vi "Record.vi"(7 "Station":string, 8 "InputResult":string, 9 "NGCode":string, 10 "PN":string, 11 "SN":string) -> (3 "Result":string)   [LabVIEW 2020]
uses:
  <vilib>/Utility/config.llb/Read Key (String).vi
  <vilib>/Utility/config.llb/Read Key (I32).vi
  <vilib>/Utility/config.llb/Write Key (String).vi
  <vilib>/Utility/config.llb/Write Key (I32).vi
  <vilib>/Utility/config.llb/NI_LVConfig.lvlib
panel:
  out "appended path":path
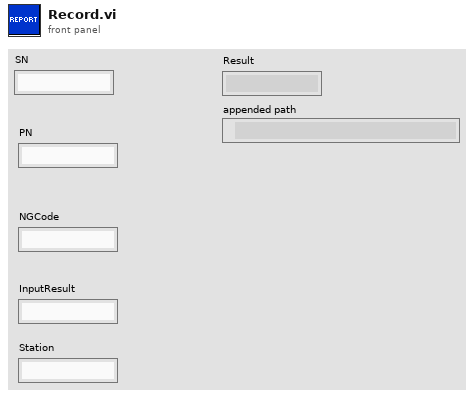
[diagram p1: front panel]
types:
  T1 = typedef "NI_LVConfig.lvlib/Config Data RefNum.ctl" = refnum<k1>
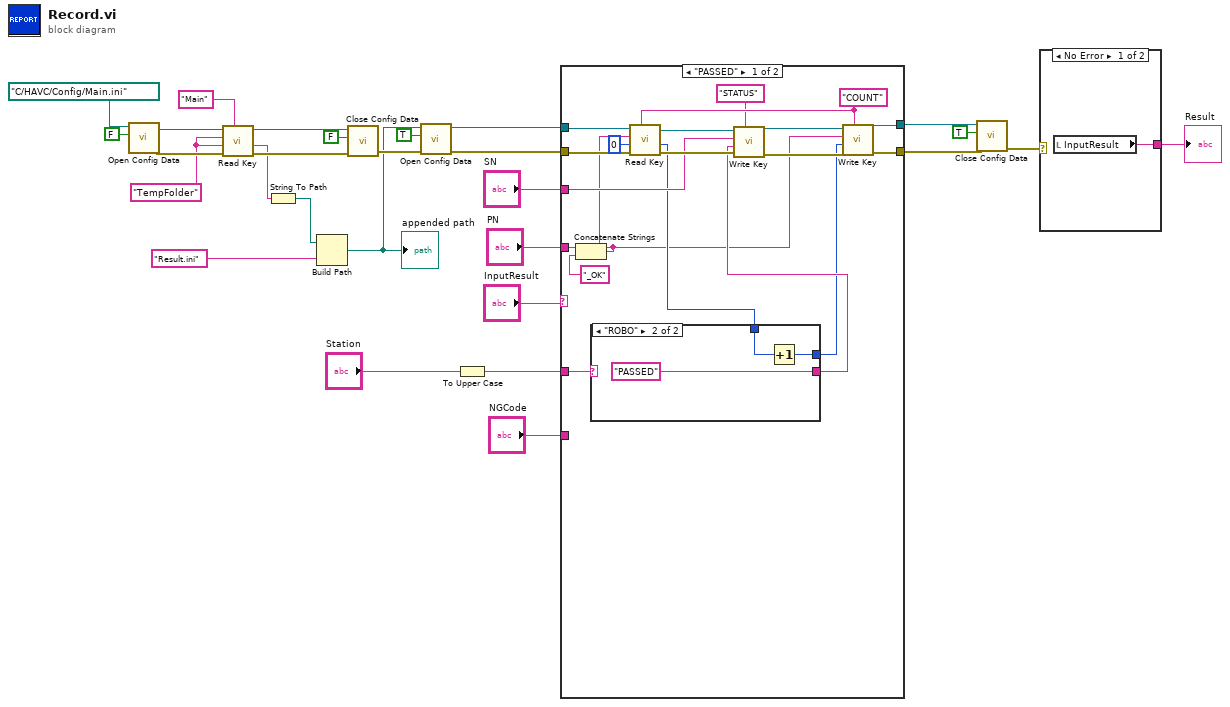
[diagram p0: block diagram]
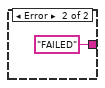
[diagram p2: hidden frame]
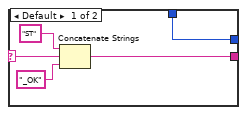
[diagram p3: hidden frame]
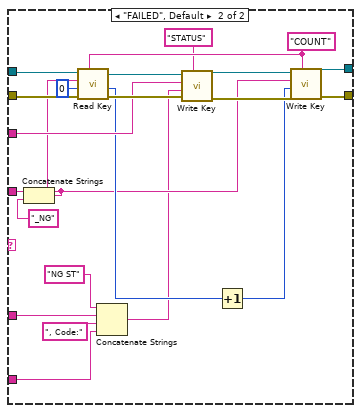
[diagram p4: hidden frame]
diagram:
  w25 = "TempFolder" ("key")
  n1 = call <vilib>:"Open Config Data.vi"("create file if necessary (T)"=FALSE, "configuration file path"=path "C:/HAVC/Config/Main.ini") -> ("error out"=w27:errorcluster, "refnum"=w26:T1)  [unwired: 7 in, 1 out]
  n2 = call-poly <vilib>:"Read Key.vi"("section"="Main", "error in (no error)"=w27, "default value"=w25, "key"=w25, "refnum"=w26) -> ("error out"=w23:errorcluster, "value"=w20:string, "refnum out"=w22:T1)  [unwired: 3 in, 1 out]
  n3 = String To Path(string=w20) -> (path=w2:path)
  n4 = Build Path(base path=w2, name or relative path="Result.ini" ("time format string (%c)")) -> (appended path=w18:path)
  "appended path" <- w18
  n5 = call <vilib>:"Close Config Data.vi"("error in (no error)"=w23, "write file if changed (T)"=FALSE, "refnum"=w22) -> ("error out"=w19:errorcluster)  [unwired: 7 in, 1 out]
  n6 = call <vilib>:"Open Config Data.vi"("error in (no error)"=w19, "create file if necessary (T)"=TRUE, "configuration file path"=w18) -> ("error out"=w14:errorcluster, "refnum"=w13:T1)  [unwired: 6 in, 1 out]
  n7 = To Upper Case(1:"Station") -> (0:w8:string)
  n8 = case shown="\"PASSED\"" "InputResult" {
    tunnel: w14 -> [w47 w77]
    tunnel: w13 -> [w46 w76]
    tunnel: [w44 w74] -> w12
    tunnel: [w45 w75] -> w11
    tunnel: "SN" -> [w36 w67]
    tunnel: w8 -> [w43 w58]
    tunnel: "PN" -> [w31 w63]
    tunnel: "NGCode" -> [_ w56]
    frame "PASSED" {
      w38 = "COUNT" ("section")
      n9 = Concatenate Strings(w31, "_OK") -> (w30:string)
      n10 = call-poly <vilib>:"Read Key.vi"("section"=w38, "error in (no error)"=w47, "default value"=0, "key"=w30, "refnum"=w46) -> ("error out"=w42:errorcluster, "value"=w33:i32, "refnum out"=w39:T1)  [unwired: 3 in, 1 out]
      n11 = case shown="\"ROBO\"" w43 {
        selector: w43 -> [w50 _]
        tunnel: [w52 "PASSED"] -> w35
        tunnel: w33 -> [w48 w53]
        tunnel: [w48 w54] -> w32
        frame Default {
          n12 = Concatenate Strings("ST", w50, "_OK" ("string")) -> (w52:string)
        }
        frame "ROBO" {
          n13 = Increment(x=w53) -> (x+1=w54:i32)
        }
      }
      n14 = call-poly <vilib>:"Write Key.vi"("section"="STATUS", "error in (no error)"=w42, "value"=w35, "key"=w36, "refnum"=w39) -> ("error out"=w41:errorcluster, "refnum out"=w40:T1)  [unwired: 4 in, 1 out]
      n15 = call-poly <vilib>:"Write Key.vi"("section"=w38, "error in (no error)"=w41, "value"=w32, "key"=w30, "refnum"=w40) -> ("error out"=w44:errorcluster, "refnum out"=w45:T1)  [unwired: 4 in, 1 out]
    }
    frame "FAILED", Default {
      w69 = "COUNT" ("section")
      n16 = Concatenate Strings(w63, "_NG") -> (w62:string)
      n17 = call-poly <vilib>:"Read Key.vi"("section"=w69, "error in (no error)"=w77, "default value"=0, "key"=w62, "refnum"=w76) -> ("error out"=w73:errorcluster, "value"=w65:i32, "refnum out"=w70:T1)  [unwired: 3 in, 1 out]
      n18 = Concatenate Strings("NG ST", w58, ", Code:" ("string"), w56) -> (w59:string)
      n19 = call-poly <vilib>:"Write Key.vi"("section"="STATUS", "error in (no error)"=w73, "value"=w59, "key"=w67, "refnum"=w70) -> ("error out"=w72:errorcluster, "refnum out"=w71:T1)  [unwired: 4 in, 1 out]
      n20 = Increment(x=w65) -> (x+1=w64:i32)
      n21 = call-poly <vilib>:"Write Key.vi"("section"=w69, "error in (no error)"=w72, "value"=w64, "key"=w62, "refnum"=w71) -> ("error out"=w74:errorcluster, "refnum out"=w75:T1)  [unwired: 4 in, 1 out]
    }
  }
  n22 = call <vilib>:"Close Config Data.vi"("error in (no error)"=w12, "write file if changed (T)"=TRUE, "refnum"=w11) -> ("error out"=w4:errorcluster)  [unwired: 7 in, 1 out]
  n23 = case shown="No Error" w4 {
    tunnel: [w78 "FAILED"] -> w3
    frame No Error {
      n24 = local read "InputResult"() -> (w78:string)
    }
    frame Error {
    }
  }
  "Result" <- w3
